vi "Read Index +1.vi"(8 "error in (no error)":errorcluster, 11 "Model_AMC in":refnum<class "Model_AMC.lvclass">) -> (0 "error out":errorcluster, 3 "Model_AMC out":refnum<class "Model_AMC.lvclass">)   [LabVIEW 2021, in "Model_AMC.lvclass"]
uses:
  Model_AMC.lvclass
  Model_AMC.lvclass/Model_AMC.ctl
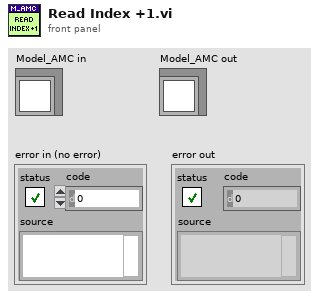
[diagram p1: front panel]
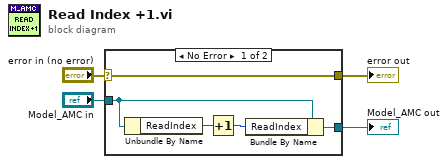
[diagram p0: block diagram]
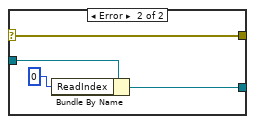
[diagram p2: hidden frame]
diagram:
  n1 = case shown="No Error" "error in (no error)" {
    selector: "error in (no error)" -> [w9 w13]
    tunnel: [w9 w13] -> w3
    tunnel: [w6 w11] -> w1
    tunnel: "Model_AMC in" -> [w7 w12]
    frame No Error {
      n2 = Unbundle By Name(w7) -> ("ReadIndex"=w8:u32)
      n3 = Increment(x=w8) -> (x+1=w5:u32)
      n4 = Bundle By Name(cluster=w7, "ReadIndex"=w5) -> (w6:refnum<class "Model_AMC.lvclass">)
    }
    frame Error {
      n5 = Bundle By Name(cluster=w12, "ReadIndex"=u32 0) -> (w11:refnum<class "Model_AMC.lvclass">)
    }
  }
  "error out" <- w3
  "Model_AMC out" <- w1
